vi "Set Valve Button States.vi"(11 "State":T1) -> ()   [LabVIEW 2015]
uses:
  System State.ctl
  Valve Button Mapping Global Action.ctl
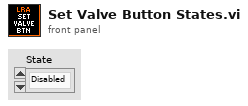
[diagram p1: front panel]
types:
  T1 = typedef "System State.ctl" = enum16{"Disabled", "E-Stop", "Standby", "Active"}
  T2 = typedef "Valve Button Mapping Global Action.ctl" = enum16{"Get", "Set"}
  T3 = typedef "Valve Name Enum.ctl" = enum16{"NV-1", "NV-2", "OV-2", "OV-3", "OV-4", "WV-2"}
  T4 = enum8{"Enabled", "Disabled", "Disabled and Grayed Out"}
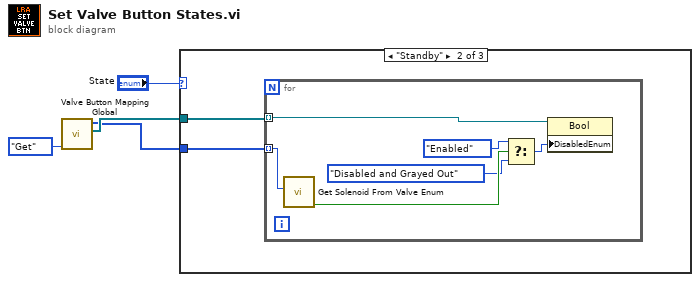
[diagram p0: block diagram]
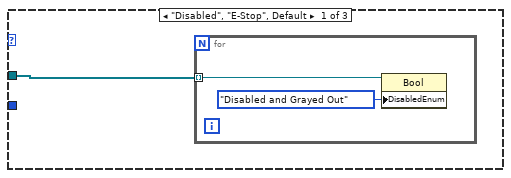
[diagram p2: hidden frame]
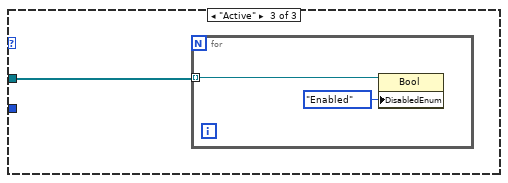
[diagram p3: hidden frame]
diagram:
  n1 = call "Valve Button Mapping Global.vi"("Action"=Valve_Button_Mapping_Global_Action."Get") -> ("Buttons"=w2:refnum<vi>[], "Valves"=w1:T3[])  [unwired: 9 in]
  n2 = case shown="\"Standby\"" "State" {
    tunnel: w2 -> [w5 w9 w16]
    tunnel: w1 -> [_ w8 _]
    frame "Disabled", "E-Stop", Default {
      n3 = for {
        tunnel: w5 -> [w7] mode=indexing
        n4 = property class="Bool"(reference=w7, "DisabledEnum"=T4."Disabled and Grayed Out" ("Disabled")) -> ()  [unwired: 1 in, 2 out]
      }
    }
    frame "Standby" {
      n5 = for {
        tunnel: w9 -> [w15] mode=indexing
        tunnel: w8 -> [w14] mode=indexing
        n6 = call "Get Solenoid From Valve Enum.vi"("Valve"=w14) -> ("Use In Standby"=w12:bool)  [unwired: 9 in, 1 out]
        n7 = Select(t=T4."Enabled" ("Disabled"), s=w12, f=T4."Disabled and Grayed Out" ("Disabled")) -> (s? t:f=w13:T4)
        n8 = property class="Bool"(reference=w15, "DisabledEnum"=w13) -> ()  [unwired: 1 in, 2 out]
      }
    }
    frame "Active" {
      n9 = for {
        tunnel: w16 -> [w18] mode=indexing
        n10 = property class="Bool"(reference=w18, "DisabledEnum"=T4."Enabled" ("Disabled")) -> ()  [unwired: 1 in, 2 out]
      }
    }
  }
